vi "Main.vi"(8 "error in (no error)":errorcluster, 11 "Process in":refnum<class "Random Process.lvclass">) -> (0 "error out":errorcluster, 3 "Process out":refnum<class "Random Process.lvclass">)   [LabVIEW 2019, in "TimingDRV Engine.lvlib" / "Random Process.lvclass"]
uses:
  Random Process.lvclass
  C:/Users/XEnderMD/Desktop/CD Project Tools/Source/Engine/Windows/Parent Classes/Process/Process.lvclass
  ee6b0e45-0e4e-4b42-bcc4-620819e24e27.vi
  Parent Classes/Process/Process.lvclass
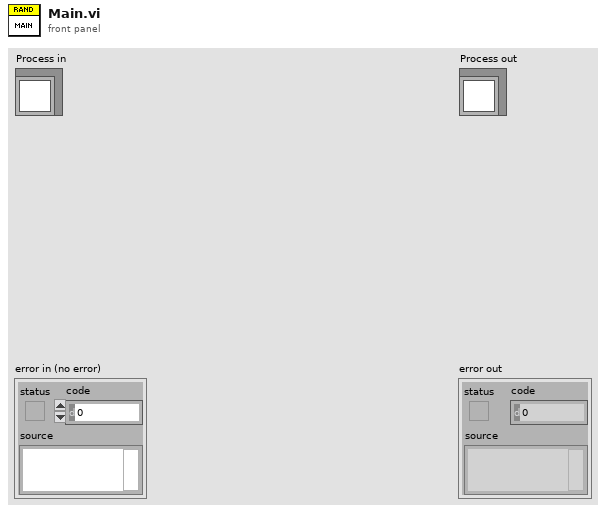
[diagram p1: front panel]
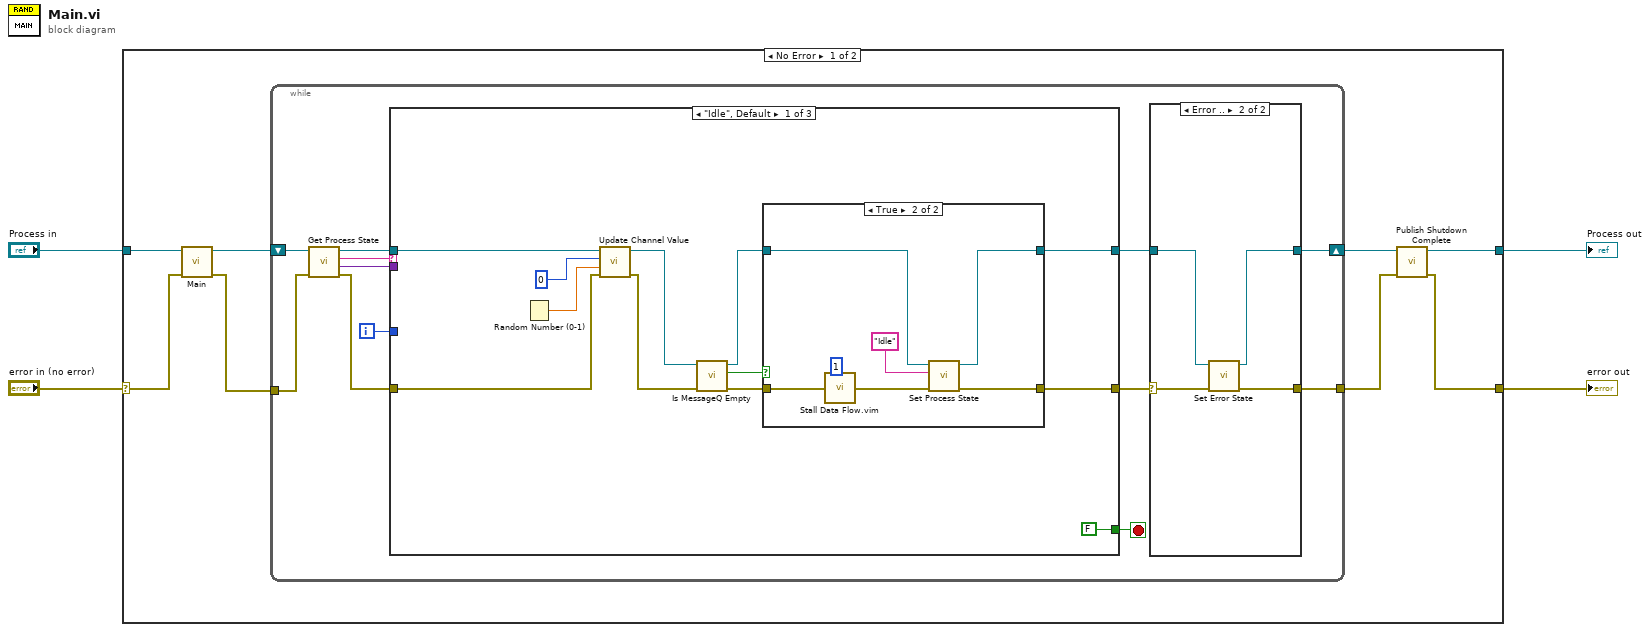
[diagram p0: block diagram]
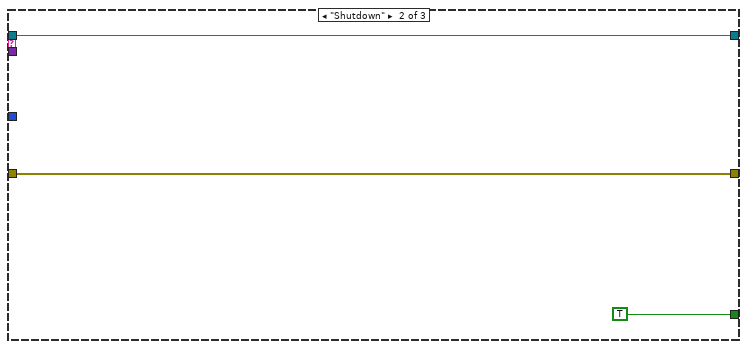
[diagram p4: hidden frame]
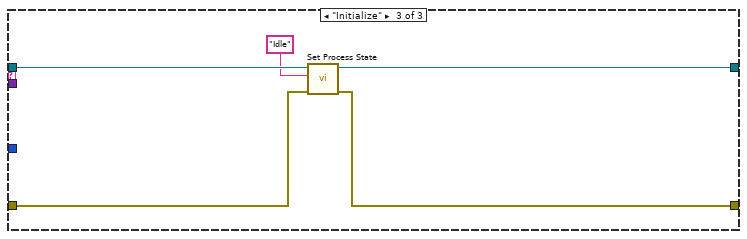
[diagram p5: hidden frame]
diagram:
  n1 = case shown="No Error" "error in (no error)" {
    selector: "error in (no error)" -> [w11 w61]
    tunnel: [w5 w61] -> w1
    tunnel: [w7 w60] -> w2
    tunnel: "Process in" -> [w12 w60]
    frame No Error {
      n2 = call-parent "Main.vi"("error in (no error)"=w11, "Process in"=w12) -> ("error out"=w9:errorcluster, "Process out"=w10:refnum<class "Random Process.lvclass">)  [unwired: 8 in]
      n3 = while {
        shift-right: [w17] -> w8
        shift-left: w10 -> [w23]
        tunnel: w9 -> [w24]
        tunnel: [w16] -> w6
        i -> [w13]
        stop <- w15 stop-if-true
        n4 = call "Get Process State.vi"("error in (no error)"=w24, "Process in"=w23) -> ("error out"=w20:errorcluster, "Payload"=w21:variant, "Command"=w14:string, "Process out"=w22:refnum<class "Random Process.lvclass">)  [unwired: 6 in]
        n5 = case shown="\"Idle\", Default" w14 {
          tunnel: w22 -> [w41 w54 w59]
          tunnel: w21 -> [_ _ _]
          tunnel: w20 -> [w40 w53 w58]
          tunnel: [w33 w54 w57] -> w19
          tunnel: [w32 w53 w56] -> w18
          tunnel: [FALSE TRUE _] -> w15
          tunnel: w13 -> [_ _ _]
          frame "Idle", Default {
            n6 = Random Number (0-1)() -> (number: 0 to 1=w31:dbl)
            n7 = call "Update Channel Value.vi"("error in (no error)"=w40, "New Value"=w31, "Channel Index"=0, "Output Process in"=w41) -> ("error out"=w38:errorcluster, "Output Process out"=w37:refnum<class "Random Process.lvclass">)  [unwired: 4 in, 2 out]
            n8 = call "Is MessageQ Empty.vi"("error in (no error)"=w38, "Process in"=w37) -> ("error out"=w35:errorcluster, "is Empty ?"=w36:bool, "Process out"=w34:refnum<class "Random Process.lvclass">)  [unwired: 7 in]
            n9 = case shown="True" w36 {
              tunnel: w35 -> [w43 w47]
              tunnel: w34 -> [w44 w50]
              tunnel: [w44 w49] -> w33
              tunnel: [w43 w48] -> w32
              frame False {
              }
              frame True {
                n10 = call "Stall Data Flow.vim"("value in"=w47, "milliseconds to wait"=u32 1) -> ("value out"=w46:errorcluster)  [unwired: 1 out]
                n11 = call "Set Process State.vi"("error in (no error)"=w46, "Command"="Idle", "Process in"=w50) -> ("error out"=w48:errorcluster, "Process out"=w49:refnum<class "Random Process.lvclass">)  [unwired: 7 in]
              }
            }
          }
          frame "Shutdown" {
          }
          frame "Initialize" {
            n12 = call "Set Process State.vi"("error in (no error)"=w58, "Command"="Idle", "Process in"=w59) -> ("error out"=w56:errorcluster, "Process out"=w57:refnum<class "Random Process.lvclass">)  [unwired: 7 in]
          }
        }
        n13 = case shown="Error .." w18 {
          selector: w18 -> [w25 w30]
          tunnel: w19 -> [w26 w29]
          tunnel: [w26 w28] -> w17
          tunnel: [w25 w27] -> w16
          frame No Error {
          }
          frame Error {
            n14 = call "Set Error State.vi"("error in (no error)"=w30, "Process in"=w29) -> ("error out"=w27:errorcluster, "Process out"=w28:refnum<class "Random Process.lvclass">)  [unwired: 8 in]
          }
        }
      }
      n15 = call "Publish Shutdown Complete.vi"("error in (no error)"=w6, "Process in"=w8) -> ("error out"=w5:errorcluster, "Process out"=w7:refnum<class "Random Process.lvclass">)  [unwired: 8 in]
    }
    frame Error {
    }
  }
  "error out" <- w1
  "Process out" <- w2
